vi "CRYUpdate Sequence Run.vi"(11 "sOption":string) -> ()   [LabVIEW 2013]
uses:
  Global/CRYCurve Library Global.vi
  CRYSystem/Data/CRYData & result stacks global.vi
  CRYSystem/Task Sequence/CRYProject Run Control Global.vi
panel:
  # "Unprotect All Data(Curves, Values,Results, Waveforms)"
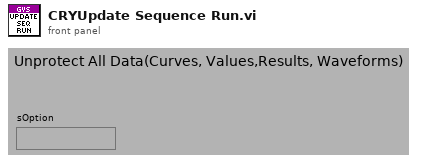
[diagram p1: front panel]
types:
  T1 = cluster{"Curve Index":i32[], "Value Index":i32[], "Result Index":i32[], "WFM Index":i32[], "Curve Names":string[], "Value Names":string[], "Result Names":string[], "WFM Names":string[]}
  T2 = cluster{"Curve OrgNames":string[], "Value OrgNames":string[], "Result OrgNames":string[], "WFM OrgNames":string[], "Curve NewNames":string[], "Value NewNames":string[], "Result NewNames":string[], "WFM NewNames":string[]}
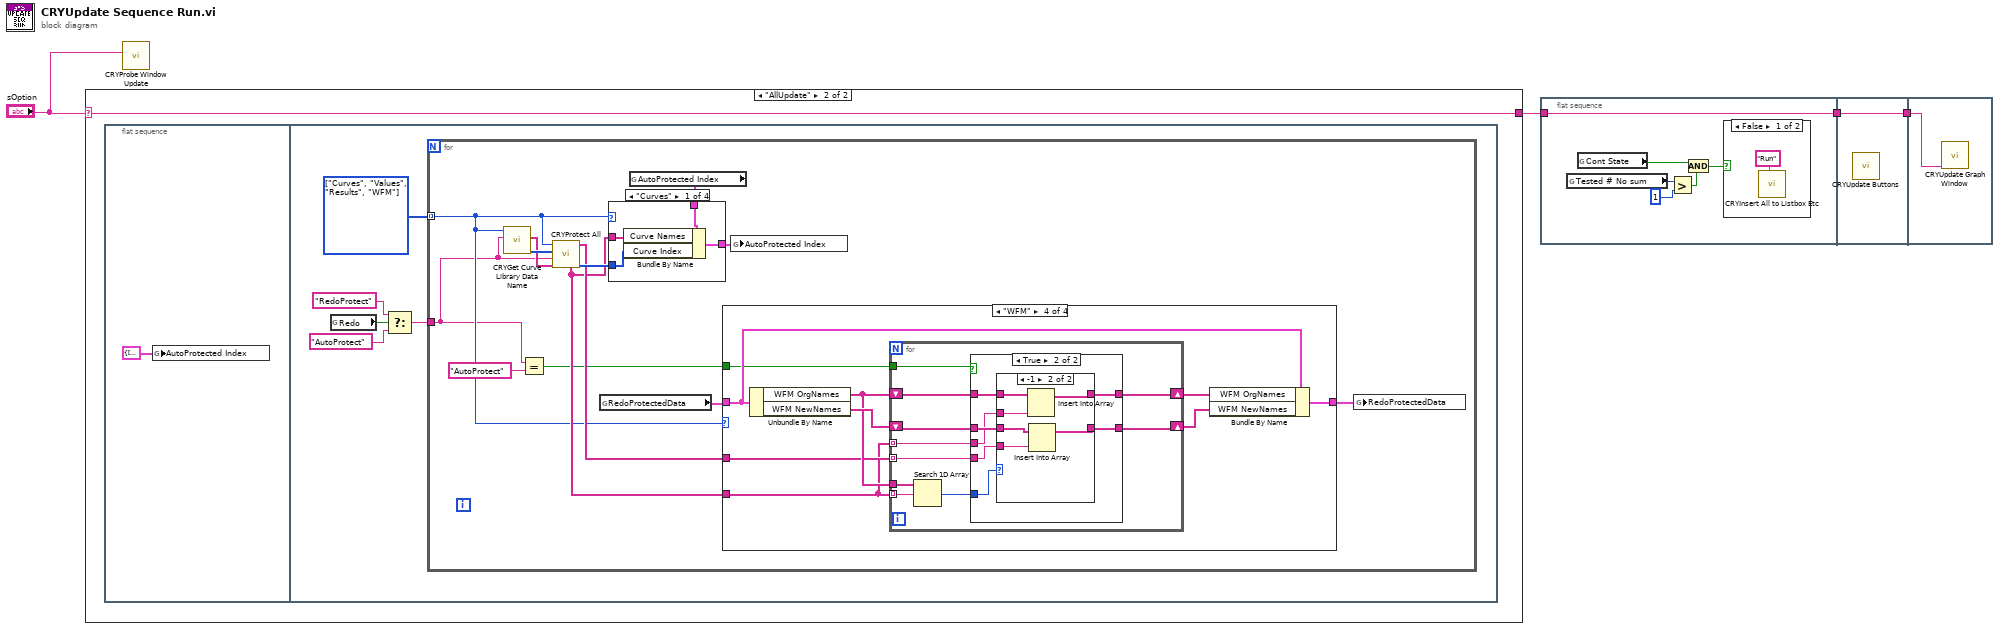
[diagram p0: block diagram]
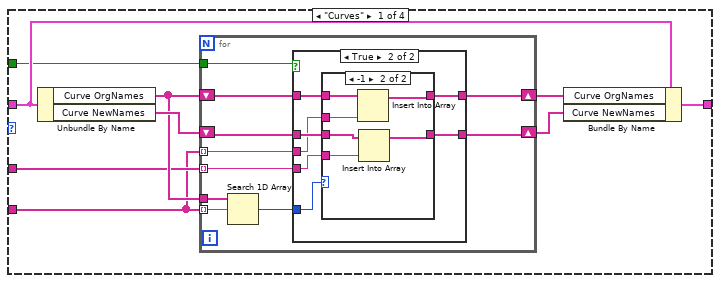
[diagram p4: hidden frame]
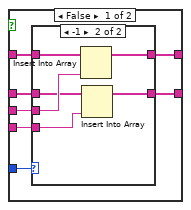
[diagram p5: hidden frame]
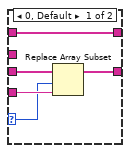
[diagram p7: hidden frame]
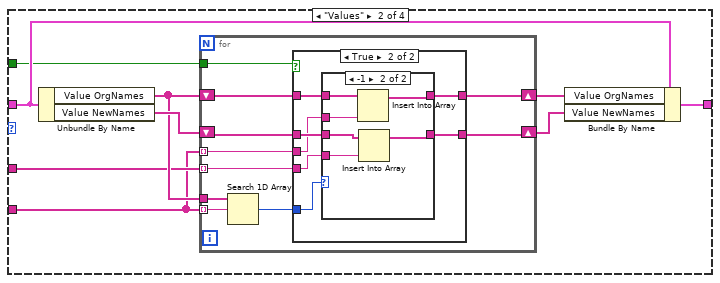
[diagram p8: hidden frame]
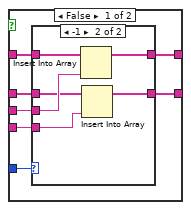
[diagram p9: hidden frame]
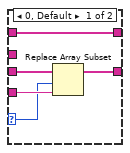
[diagram p11: hidden frame]
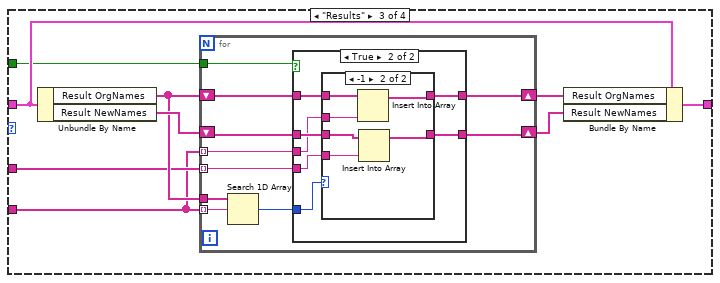
[diagram p12: hidden frame]
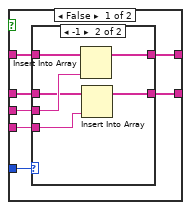
[diagram p13: hidden frame]
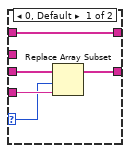
[diagram p15: hidden frame]
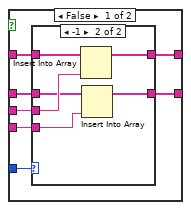
[diagram p16: hidden frame]
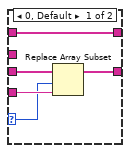
[diagram p18: hidden frame]
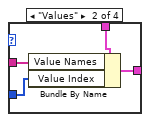
[diagram p19: hidden frame]
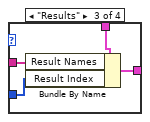
[diagram p20: hidden frame]
diagram:
  n1 = case shown="\"AllUpdate\"" "sOption" {
    selector: "sOption" -> [w5 w6]
    tunnel: [w5 w6] -> w3
    frame "SubSequenceRemoveUpdate", Default {
    }
    frame "AllUpdate" {
      n2 = flat-sequence {
        frame #0 {
          n3 = global write "CRYCurve Library Global.vi" "AutoProtected Index"(T1 {"Curve Index"=[], "Value Index"=[], "Result Index"=[], "WFM Index"=[], "Curve Names"=[], "Value Names"=[], "Result Names"=[], "WFM Names"=[]} ("AutoProtected Index")) -> ()
        }
        frame #1 {
          w8 = enum16{"Curves", "Values", "Results", "WFM"}[] [enum."Curves", enum."Values", enum."Results", enum."WFM"] items=["Curves", "Values", "Results", "WFM"]
          n4 = global read "CRYData & result stacks global.vi" "Redo"() -> (w9:bool)
          n5 = Select(t="RedoProtect", s=w9, f="AutoProtect") -> (s? t:f=w10:string)
          n6 = for {
            tunnel: w8 -> [w16] mode=indexing
            tunnel: w10 -> [w15]
            n7 = call "CRYGet Curve Library Data Name.vi"("sAction"=w15, "Type"=w16) -> ("Index"=w25:i32[], "sNames"=w21:string[])  [unwired: 6 in, 2 out]
            n8 = Equal?(x=w15, y="AutoProtect") -> (x = y?=w13:bool)
            n9 = call "CRYProtect All.vi"("sNames"=w21, "sOption"=w15, "Index"=w25, "Type"=w16) -> ("Inserted Index"=w22:i32[], "Protected NewNames"=w18:string[], "Protected OrgNames"=w17:string[])  [unwired: 3 in, 2 out]
            n10 = global read "CRYCurve Library Global.vi" "RedoProtectedData"() -> (w20:T2)
            n11 = global read "CRYCurve Library Global.vi" "AutoProtected Index"() -> (w23:T1)
            n12 = case shown="\"Curves\"" w16 {
              tunnel: w23 -> [w237 w241 w245 w249]
              tunnel: [w236 w240 w244 w248] -> w24
              tunnel: w22 -> [w234 w238 w242 w246]
              tunnel: w17 -> [w235 w239 w243 w247]
              frame "Curves" {
                n13 = Bundle By Name(cluster=w237, "Curve Names"=w235, "Curve Index"=w234) -> (w236:T1)
              }
              frame "Values" {
                n14 = Bundle By Name(cluster=w241, "Value Names"=w239, "Value Index"=w238) -> (w240:T1)
              }
              frame "Results" {
                n15 = Bundle By Name(cluster=w245, "Result Names"=w243, "Result Index"=w242) -> (w244:T1)
              }
              frame "WFM" {
                n16 = Bundle By Name(cluster=w249, "WFM Names"=w247, "WFM Index"=w246) -> (w248:T1)
              }
            }
            n17 = case shown="\"WFM\"" w16 {
              tunnel: w20 -> [w34 w86 w138 w190]
              tunnel: [w33 w85 w137 w189] -> w19
              tunnel: w18 -> [w28 w80 w132 w184]
              tunnel: w17 -> [w27 w79 w131 w183]
              tunnel: w13 -> [w26 w78 w130 w182]
              frame "Curves" {
                n18 = Unbundle By Name(w34) -> ("Curve OrgNames"=w29:string[], "Curve NewNames"=w30:string[])
                n19 = for {
                  tunnel: w29 -> [w38]
                  tunnel: w28 -> [w41] mode=indexing
                  tunnel: w27 -> [w44] mode=indexing
                  shift-right: [w42] -> w32
                  shift-left: w29 -> [w43]
                  shift-right: [w39] -> w31
                  shift-left: w30 -> [w40]
                  tunnel: w27 -> [w37] mode=indexing
                  tunnel: w26 -> [w35]
                  n20 = Search 1D Array(1D array=w38, element=w37) -> (index of element=w36:i32)  [unwired: 1 in]
                  n21 = case shown="True" w35 {
                    tunnel: w44 -> [w51 w60]
                    tunnel: w43 -> [w50 w62]
                    tunnel: [w49 w61] -> w42
                    tunnel: w41 -> [w48 w64]
                    tunnel: w40 -> [w47 w66]
                    tunnel: [w46 w65] -> w39
                    tunnel: w36 -> [w45 w63]
                    frame False {
                      n22 = case shown="-1" w45 {
                        tunnel: w51 -> [_ w57]
                        tunnel: w50 -> [w53 w59]
                        tunnel: [w53 w58] -> w49
                        tunnel: w48 -> [_ w56]
                        tunnel: w47 -> [w52 w55]
                        tunnel: [w52 w54] -> w46
                        frame 0, Default {
                        }
                        frame -1 {
                          n23 = Insert Into Array(array=w59, new element=w57) -> (w58:string[])  [unwired: 1 in]
                          n24 = Insert Into Array(array=w55, new element=w56) -> (w54:string[])  [unwired: 1 in]
                        }
                      }
                    }
                    frame True {
                      n25 = case shown="-1" w63 {
                        selector: w63 -> [w67 _]
                        tunnel: w66 -> [w71 w75]
                        tunnel: [w70 w74] -> w65
                        tunnel: w64 -> [w69 w73]
                        tunnel: w62 -> [w68 w77]
                        tunnel: [w68 w76] -> w61
                        tunnel: w60 -> [_ w72]
                        frame 0, Default {
                          n26 = Replace Array Subset(array=w71, new element=w69, index=w67) -> (w70:string[])
                        }
                        frame -1 {
                          n27 = Insert Into Array(array=w77, new element=w72) -> (w76:string[])  [unwired: 1 in]
                          n28 = Insert Into Array(array=w75, new element=w73) -> (w74:string[])  [unwired: 1 in]
                        }
                      }
                    }
                  }
                }
                n29 = Bundle By Name(cluster=w34, "Curve OrgNames"=w32, "Curve NewNames"=w31) -> (w33:T2)
              }
              frame "Values" {
                n30 = Unbundle By Name(w86) -> ("Value OrgNames"=w81:string[], "Value NewNames"=w82:string[])
                n31 = for {
                  tunnel: w81 -> [w90]
                  tunnel: w80 -> [w93] mode=indexing
                  tunnel: w79 -> [w96] mode=indexing
                  shift-right: [w94] -> w84
                  shift-left: w81 -> [w95]
                  shift-right: [w91] -> w83
                  shift-left: w82 -> [w92]
                  tunnel: w79 -> [w89] mode=indexing
                  tunnel: w78 -> [w87]
                  n32 = Search 1D Array(1D array=w90, element=w89) -> (index of element=w88:i32)  [unwired: 1 in]
                  n33 = case shown="True" w87 {
                    tunnel: w96 -> [w103 w112]
                    tunnel: w95 -> [w102 w114]
                    tunnel: [w101 w113] -> w94
                    tunnel: w93 -> [w100 w116]
                    tunnel: w92 -> [w99 w118]
                    tunnel: [w98 w117] -> w91
                    tunnel: w88 -> [w97 w115]
                    frame False {
                      n34 = case shown="-1" w97 {
                        tunnel: w103 -> [_ w109]
                        tunnel: w102 -> [w105 w111]
                        tunnel: [w105 w110] -> w101
                        tunnel: w100 -> [_ w108]
                        tunnel: w99 -> [w104 w107]
                        tunnel: [w104 w106] -> w98
                        frame 0, Default {
                        }
                        frame -1 {
                          n35 = Insert Into Array(array=w111, new element=w109) -> (w110:string[])  [unwired: 1 in]
                          n36 = Insert Into Array(array=w107, new element=w108) -> (w106:string[])  [unwired: 1 in]
                        }
                      }
                    }
                    frame True {
                      n37 = case shown="-1" w115 {
                        selector: w115 -> [w119 _]
                        tunnel: w118 -> [w123 w127]
                        tunnel: [w122 w126] -> w117
                        tunnel: w116 -> [w121 w125]
                        tunnel: w114 -> [w120 w129]
                        tunnel: [w120 w128] -> w113
                        tunnel: w112 -> [_ w124]
                        frame 0, Default {
                          n38 = Replace Array Subset(array=w123, new element=w121, index=w119) -> (w122:string[])
                        }
                        frame -1 {
                          n39 = Insert Into Array(array=w129, new element=w124) -> (w128:string[])  [unwired: 1 in]
                          n40 = Insert Into Array(array=w127, new element=w125) -> (w126:string[])  [unwired: 1 in]
                        }
                      }
                    }
                  }
                }
                n41 = Bundle By Name(cluster=w86, "Value OrgNames"=w84, "Value NewNames"=w83) -> (w85:T2)
              }
              frame "Results" {
                n42 = Unbundle By Name(w138) -> ("Result OrgNames"=w133:string[], "Result NewNames"=w134:string[])
                n43 = for {
                  tunnel: w133 -> [w142]
                  tunnel: w132 -> [w145] mode=indexing
                  tunnel: w131 -> [w148] mode=indexing
                  shift-right: [w146] -> w136
                  shift-left: w133 -> [w147]
                  shift-right: [w143] -> w135
                  shift-left: w134 -> [w144]
                  tunnel: w131 -> [w141] mode=indexing
                  tunnel: w130 -> [w139]
                  n44 = Search 1D Array(1D array=w142, element=w141) -> (index of element=w140:i32)  [unwired: 1 in]
                  n45 = case shown="True" w139 {
                    tunnel: w148 -> [w155 w164]
                    tunnel: w147 -> [w154 w166]
                    tunnel: [w153 w165] -> w146
                    tunnel: w145 -> [w152 w168]
                    tunnel: w144 -> [w151 w170]
                    tunnel: [w150 w169] -> w143
                    tunnel: w140 -> [w149 w167]
                    frame False {
                      n46 = case shown="-1" w149 {
                        tunnel: w155 -> [_ w161]
                        tunnel: w154 -> [w157 w163]
                        tunnel: [w157 w162] -> w153
                        tunnel: w152 -> [_ w160]
                        tunnel: w151 -> [w156 w159]
                        tunnel: [w156 w158] -> w150
                        frame 0, Default {
                        }
                        frame -1 {
                          n47 = Insert Into Array(array=w163, new element=w161) -> (w162:string[])  [unwired: 1 in]
                          n48 = Insert Into Array(array=w159, new element=w160) -> (w158:string[])  [unwired: 1 in]
                        }
                      }
                    }
                    frame True {
                      n49 = case shown="-1" w167 {
                        selector: w167 -> [w171 _]
                        tunnel: w170 -> [w175 w179]
                        tunnel: [w174 w178] -> w169
                        tunnel: w168 -> [w173 w177]
                        tunnel: w166 -> [w172 w181]
                        tunnel: [w172 w180] -> w165
                        tunnel: w164 -> [_ w176]
                        frame 0, Default {
                          n50 = Replace Array Subset(array=w175, new element=w173, index=w171) -> (w174:string[])
                        }
                        frame -1 {
                          n51 = Insert Into Array(array=w181, new element=w176) -> (w180:string[])  [unwired: 1 in]
                          n52 = Insert Into Array(array=w179, new element=w177) -> (w178:string[])  [unwired: 1 in]
                        }
                      }
                    }
                  }
                }
                n53 = Bundle By Name(cluster=w138, "Result OrgNames"=w136, "Result NewNames"=w135) -> (w137:T2)
              }
              frame "WFM" {
                n54 = Unbundle By Name(w190) -> ("WFM OrgNames"=w185:string[], "WFM NewNames"=w186:string[])
                n55 = for {
                  tunnel: w185 -> [w194]
                  tunnel: w184 -> [w197] mode=indexing
                  tunnel: w183 -> [w200] mode=indexing
                  shift-right: [w198] -> w188
                  shift-left: w185 -> [w199]
                  shift-right: [w195] -> w187
                  shift-left: w186 -> [w196]
                  tunnel: w183 -> [w193] mode=indexing
                  tunnel: w182 -> [w191]
                  n56 = Search 1D Array(1D array=w194, element=w193) -> (index of element=w192:i32)  [unwired: 1 in]
                  n57 = case shown="True" w191 {
                    tunnel: w200 -> [w207 w216]
                    tunnel: w199 -> [w206 w218]
                    tunnel: [w205 w217] -> w198
                    tunnel: w197 -> [w204 w220]
                    tunnel: w196 -> [w203 w222]
                    tunnel: [w202 w221] -> w195
                    tunnel: w192 -> [w201 w219]
                    frame False {
                      n58 = case shown="-1" w201 {
                        tunnel: w207 -> [_ w213]
                        tunnel: w206 -> [w209 w215]
                        tunnel: [w209 w214] -> w205
                        tunnel: w204 -> [_ w212]
                        tunnel: w203 -> [w208 w211]
                        tunnel: [w208 w210] -> w202
                        frame 0, Default {
                        }
                        frame -1 {
                          n59 = Insert Into Array(array=w215, new element=w213) -> (w214:string[])  [unwired: 1 in]
                          n60 = Insert Into Array(array=w211, new element=w212) -> (w210:string[])  [unwired: 1 in]
                        }
                      }
                    }
                    frame True {
                      n61 = case shown="-1" w219 {
                        selector: w219 -> [w223 _]
                        tunnel: w222 -> [w227 w231]
                        tunnel: [w226 w230] -> w221
                        tunnel: w220 -> [w225 w229]
                        tunnel: w218 -> [w224 w233]
                        tunnel: [w224 w232] -> w217
                        tunnel: w216 -> [_ w228]
                        frame 0, Default {
                          n62 = Replace Array Subset(array=w227, new element=w225, index=w223) -> (w226:string[])
                        }
                        frame -1 {
                          n63 = Insert Into Array(array=w233, new element=w228) -> (w232:string[])  [unwired: 1 in]
                          n64 = Insert Into Array(array=w231, new element=w229) -> (w230:string[])  [unwired: 1 in]
                        }
                      }
                    }
                  }
                }
                n65 = Bundle By Name(cluster=w190, "WFM OrgNames"=w188, "WFM NewNames"=w187) -> (w189:T2)
              }
            }
            n66 = global write "CRYCurve Library Global.vi" "AutoProtected Index"(w24) -> ()
            n67 = global write "CRYCurve Library Global.vi" "RedoProtectedData"(w19) -> ()
          }
        }
      }
    }
  }
  n68 = call "CRYProbe Window Update.vi"("sAction"="sOption") -> ()  [unwired: 11 in]
  n69 = flat-sequence {
    tunnel: [w255] -> w2
    tunnel: w3 -> [w255]
    tunnel: [w257] -> w1
    tunnel: w2 -> [w257]
    tunnel: w1 -> [w258]
    frame #0 {
      n70 = global read "CRYData & result stacks global.vi" "Tested # No sum"() -> (w253:u16)
      n71 = global read "CRYProject Run Control Global.vi" "Cont State"() -> (w252:bool)
      n72 = Greater?(x=w253, y=u16 1) -> (0:w251:bool)
      n73 = And(x=w252, y=w251) -> (x .and. y?=w250:bool)
      n74 = case shown="False" w250 {
        frame False {
          n75 = call "CRYInsert All to Listbox Etc.vi"("sAction"="Run") -> ()  [unwired: 11 in]
        }
        frame True {
        }
      }
    }
    frame #1 {
      n76 = call "CRYUpdate Buttons.vi"() -> ()  [unwired: 1 in, 11 out]
    }
    frame #2 {
      n77 = call "CRYUpdate Graph Window.vi"("sOption"=w258) -> ()  [unwired: 4 in, 7 out]
    }
  }
